vi "MTM2_getSample_temperaturesMeasured.vi"(8 "error in (no error)":errorcluster, 11 "temperaturesMeasured_Ctl":T1={"temps[72]"=[0.0, 0.0, 0.0, 0.0, 0.0, 0.0, 0.0, 0.0, 0.0, 0.0, 0.0, 0.0, 0.0, 0.0, 0.0, 0.0, 0.0, 0.0, 0.0, 0.0, 0.0, 0.0, 0.0, 0.0, 0.0, 0.0, 0.0, 0.0, 0.0, 0.0, 0.0, 0.0, 0.0, 0.0, 0.0, 0.0, 0.0, 0.0, 0.0, 0.0, 0.0, 0.0, 0.0, 0.0, 0.0, 0.0, 0.0, 0.0, 0.0, 0.0, 0.0, 0.0, 0.0, 0.0, 0.0, 0.0, 0.0, 0.0, 0.0, 0.0, 0.0, 0.0, 0.0, 0.0, 0.0, 0.0, 0.0, 0.0, 0.0, 0.0, 0.0, 0.0], "intakeTemperatures[4]"=[0.0, 0.0, 0.0, 0.0], "exhaustTemperatures[4]"=[0.0, 0.0, 0.0, 0.0]}) -> (0 "error out":errorcluster, 2 "function return":i32, 3 "temperaturesMeasured_Ctl out":T1)   [LabVIEW 2018, in "SALLV_MTM2.lvlib"]
doc: "int MTM2_shm_getSample_temperaturesMeasuredLV(MTM2_temperaturesMeasuredLV *temperaturesMeasured_Ctl );"
uses:
  SALLV_MTM2.lvlib
  DataTypes/temperaturesMeasured.ctl
  SALLV_MTM2.so
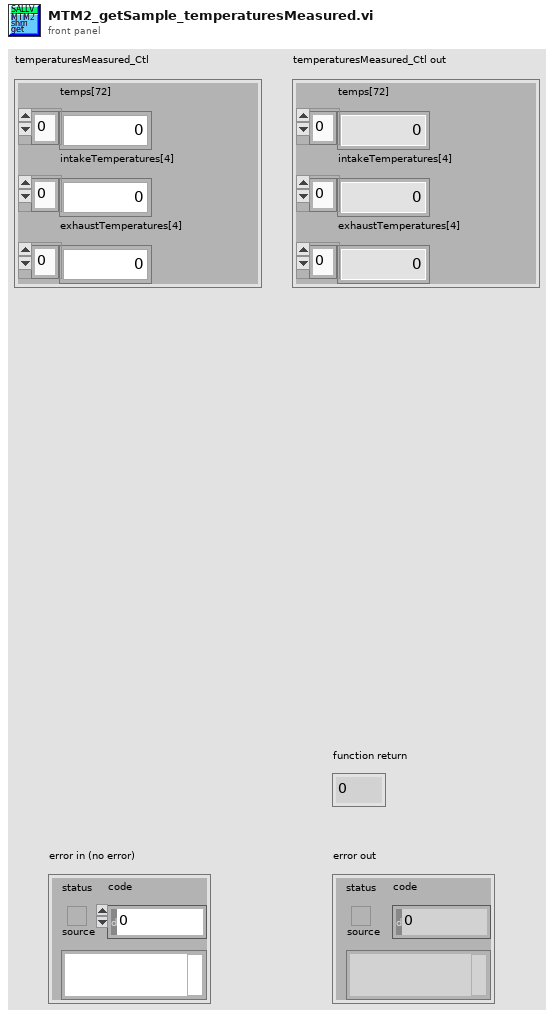
[diagram p1: front panel]
types:
  T1 = typedef "SALLV_MTM2.lvlib/temperaturesMeasured.ctl" = cluster{"temps[72]":dbl[], "intakeTemperatures[4]":dbl[], "exhaustTemperatures[4]":dbl[]}
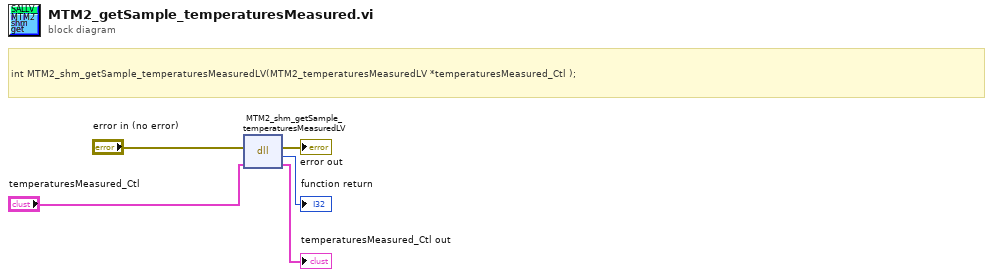
[diagram p0: block diagram]
diagram:
  # "int MTM2_shm_getSample_temperaturesMeasuredLV(MTM2_temperaturesMeasuredLV *temperaturesMeasured_Ctl );"
  n1 = dll-call lib="home/ttsai/Document/salApiMTM2/SALLV_MTM2/SALLV_MTM2.*" fn="MTM2_shm_getSample_temperaturesMeasuredLV"(error in="error in (no error)", "temperaturesMeasured_Ctl"="temperaturesMeasured_Ctl") -> (error out=→"error out":errorcluster, →"function return":i32, "temperaturesMeasured_Ctl"=→"temperaturesMeasured_Ctl out":T1)  [unwired: 2 in, 1 out]
